vi "general_measurement_KT_2.vi"(9 "Measurement Data":dbl[](array[numeric]), 10 "Array 4":dbl[](array[numeric]), 11 "Array 3":dbl[](array[numeric])) -> (1 "Measurement":T1, 2 "Array":dbl[](array[numeric]), 3 "Array 2":dbl[](array[numeric]), 4 "Array 5":dbl[](array[numeric]), 5 "Seebeck coefficient":cluster{"Y":dbl[], "Y":dbl[]}[](graph))   [LabVIEW 2011]
uses:
  <vilib>/express/express arith-compare/Formula/XNode/ExpressFormulaBlockNode.xnode
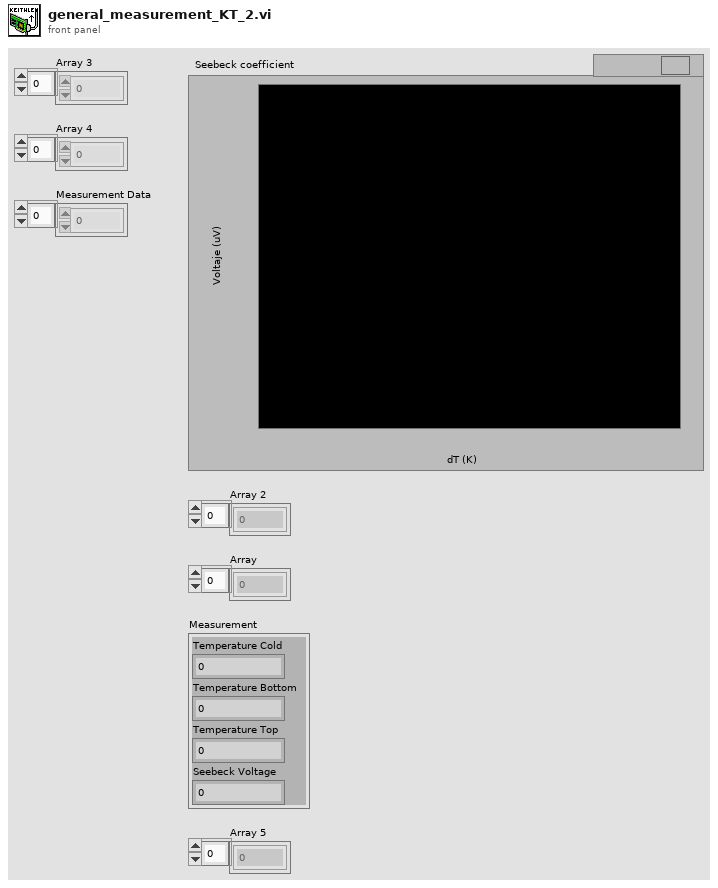
[diagram p1: front panel]
types:
  T1 = cluster{"Temperature Cold":dbl, "Temperature Bottom":dbl, "Temperature Top":dbl, "Seebeck Voltage":dbl}
  T2 = cluster{"Measurement Data[0]":dbl, "Measurement Data[1]":dbl, "Measurement Data[2]":dbl, "Measurement Data[3]":dbl, "Measurement Data[4]":dbl, "Measurement Data[5]":dbl, "Measurement Data[6]":dbl, "Measurement Data[7]":dbl, "Measurement Data[8]":dbl}
  T3 = cluster{"Result":dbl, "Result":dbl, "Result":dbl, "Measurement Data[3]":dbl}
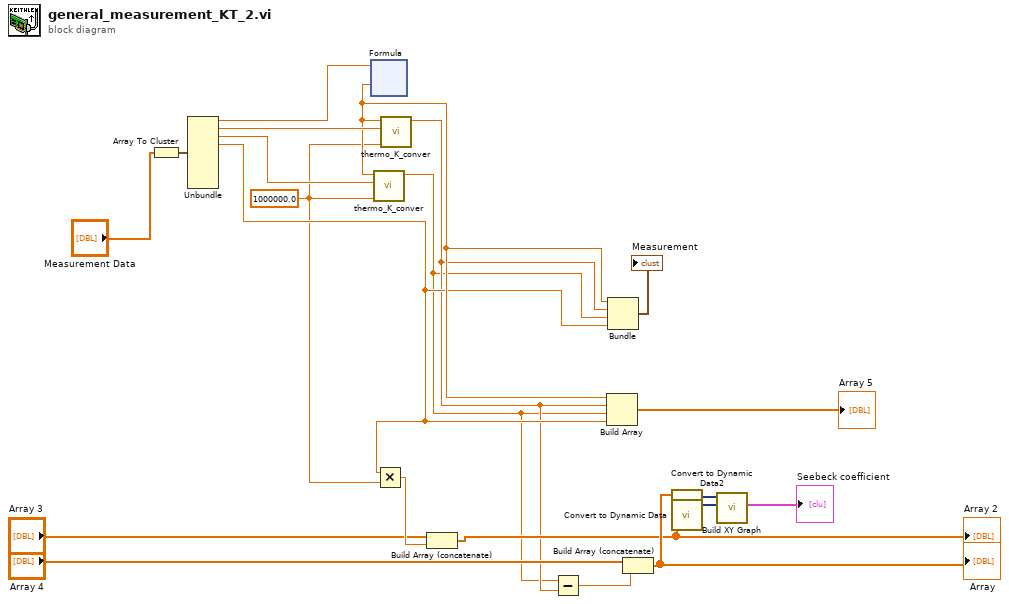
[diagram p0: block diagram]
diagram:
  w1 = 1000000.0 ("y")
  n1 = Array To Cluster(array="Measurement Data") -> (cluster=w6:T2)
  n2 = Unbundle(w6) -> ("Measurement Data[0]"=w12:dbl, "Measurement Data[1]"=w9:dbl, "Measurement Data[2]"=w10:dbl, "Measurement Data[3]"=w4:dbl)  [unwired: 5 out]
  n3 = xnode ("Formula")("R"=w12) -> ("Result"=w5:dbl)  [unwired: 1 in, 1 out]
  n4 = call "thermo_K_conver.vi"("y"=w1, "Measurement Data[1]"=w10, "Measurement Data[0]"=w5) -> ("Result"=w2:dbl)  [unwired: 8 in]
  n5 = Multiply(x=w4, y=w1) -> (x*y=w21:dbl)
  n6 = call "thermo_K_conver.vi"("y"=w1, "Measurement Data[1]"=w9, "Measurement Data[0]"=w5) -> ("Result"=w3:dbl)  [unwired: 8 in]
  n7 = Build Array (concatenate)("Array 3", w21) -> (w17:dbl[])
  "Array 2" <- w17
  n8 = Subtract(x=w2, y=w3) -> (x-y=w15:dbl)
  n9 = Build Array(w5, w3, w2, w4) -> (→"Array 5":dbl[])
  n10 = Bundle("Result"=w5, "Result"=w3, "Result"=w2, "Measurement Data[3]"=w4) -> (→"Measurement":T3)  [unwired: 1 in]
  n11 = Build Array (concatenate)("Array 4", w15) -> (w19:dbl[])
  "Array" <- w19
  n12 = call "Convert to Dynamic Data2"("Array"=w19) -> ("Dynamic Data Type"=w20:dynamicdata)  [unwired: 3 in]
  n13 = call "Convert to Dynamic Data"("Array"=w17) -> ("Dynamic Data Type"=w18:dynamicdata)  [unwired: 3 in]
  n14 = call "Build XY Graph"("Y Input"=w18, "X Input"=w20) -> ("XY Graph"=→"Seebeck coefficient":cluster{"Y":dbl[], "Y":dbl[]}[])  [unwired: 3 in, 6 out]
